vi "Daten zu cRIO.vi"   [LabVIEW 2020, in "Kommunikation mit PC.lvlib"]
uses:
  Kommunikation mit PC.lvlib
  Regler/Druckregler/Aktionen Param. Druckregler.ctl
  Allgemein/Aktionen FGV Dichtheitstest.ctl
  Allgemein/FGV Zustaende Aktionen.ctl
  Stoermeldungen/FGV Stoerungen Aktionen.ctl
  Verwaltung/FGV OUT Aktionen.ctl
  Allgemein/FGV FT-IR Kuehlung Aktionen.ctl
  Allgemein/Aktion FGV Klima.ctl
  Allgemein/Aktion FGV T90.ctl
  Allgemein/FGV Analysator aktiv.ctl
  Allgemein/Aktion FGV Zustandsbeleuchtung schalten.ctl
  Allgemein/Cluster Komm Systemeinstellungen.ctl
  Allgemein/Aktion FGV Komm Systemeinstellungen.ctl
  Konfig-Dateien/FGV Betriebsdaten Aktionen.ctl
  Konfig-Dateien/Aktionen Konfig.ctl
  Konfig-Dateien/Konfig-Dateien.lvlib
  Regler/Druckregler/Druckregler.lvlib
  Allgemein/Allgemein.lvlib
  Stoermeldungen/Stoermeldungen.lvlib
  Verwaltung/Verwaltung - cRIO.lvlib
  SysLog/SysLog_cRIO.lvlib
  CAN Interface/CAN Interface.lvlib
  CAN Interface/FGV CAN Daten Aktionen.ctl
  CAN Interface/Baude Rate.ctl
  Seiten/CAN Konfig/Konfig Daten PC.ctl
  Seiten/CAN Konfig/CAN Konfig.lvlib
types:
  T1 = typedef "Allgemein.lvlib/Aktion FGV Komm Systemeinstellungen.ctl" = enum16{"lesen", "schreiben"}
  T2 = typedef "Allgemein.lvlib/Cluster Komm Systemeinstellungen.ctl" = cluster{"ECO LNG":bool}
  T3 = typedef "Allgemein.lvlib/Aktion FGV Zustandsbeleuchtung schalten.ctl" = enum16{"lesen", "prüfen", "init", "Bit löschen", "ansteuern", "Aufheizphase"}
  T4 = typedef "Allgemein.lvlib/FGV Analysator aktiv.ctl" = enum16{"lesen", "Analysator", "CG Aufschaltung", "KAL Zustand", "AutaKal GT?"}
  T5 = typedef "Allgemein.lvlib/FGV Zustaende Aktionen.ctl" = enum16{"lesen", "Zustand PC", "Zustand cRIO", "Bildnummer", "Samplepoint", "Sysloglevel"}
  T6 = typedef "Allgemein.lvlib/Aktion FGV T90.ctl" = enum16{"lesen", "schreiben"}
  T7 = typedef "Allgemein.lvlib/Aktion FGV Klima.ctl" = enum16{"lesen", "Klimaanlage", "Container", "PNS"}
  T8 = typedef "Allgemein.lvlib/FGV FT-IR Kuehlung Aktionen.ctl" = enum16{"lesen", "Kühlung?"}
  T9 = typedef "Verwaltung - cRIO.lvlib/FGV OUT Aktionen.ctl" = enum16{"lesen", "ANA OUT", "DO 0-31", "DO 32-47"}
  T10 = typedef "Stoermeldungen.lvlib/FGV Stoerungen Aktionen.ctl" = enum16{"lesen", "Störung aktiv?", "1-64", "65-128"}
  T11 = typedef "Allgemein.lvlib/Aktionen FGV Dichtheitstest.ctl" = enum16{"lesen", "schreiben"}
  T12 = typedef "Regler.lvlib/Druckregler.lvlib/Aktionen Param. Druckregler.ctl" = enum16{"lesen", "schreiben", "Regler FT-IR", "Regler Ausgang", "Regler Durchfluss", "Regler PMA", "Regler NDIR", "Regler Filterblock", "Regler Gaskühler", "Regler Kalter Block"}
  T13 = typedef "Bildwechsel.lvlib/Bild-Auswahl.ctl" = enum16{"lesen", "Initialisieren", "Beenden", "Grafik", "Anlagenübersicht", "Anlagengrenzwerte", "Log Konfig", "Gaszuordnung AO", "Erw. Konfiguration", "FT-IR  ", "Störmeldungen", "Störmeldepuffer", "Störmeldekonfig", "PNS Grenzwerte", "Statusübersicht", "Linearisierung", "ARN", "EPA Dichtheitstest", "FID", "PMA", "CalGas", "Lambda", "Interference", "Amium PNS", "EPA T90", "Interference N2O", "Scheduler", "Systemeinstellungen", "EPA Drift", "CAN Konfig"}
  T14 = cluster{"SysLogLevel":u16, "Software Version":string}
  T15 = cluster{"Numeric":u16, "Numeric":u16, "Numeric":u16, "Numeric":u16, "Numeric":u16}
  T16 = cluster{"Numeric":u16, "Numeric":u16, "Numeric":u16}
  T17 = cluster{"Boolean":bool, "Boolean":bool, "Boolean":bool}
  T18 = typedef "Konfig-Dateien.lvlib/FGV Betriebsdaten Aktionen.ctl" = enum16{"lesen", "Anlagengrenzw.", "PID Param.", "Sonstige", "Sensor Para."}
  T19 = typedef "Konfig-Dateien.lvlib/Aktionen Konfig.ctl" = enum16{"lesen", "laden", "speichern  System.ini", "speichern Anlagengrenzw.", "speichern PID + Sonstige", "speichern BSZ BMP", "speichern BSZ FT-IR", "speichern Stickstoff Bef.", "speichern Ext. Stickstoff Bef.", "speichern CAN_Konfig"}
  T20 = typedef "CAN Konfig.lvlib/Konfig Daten PC.ctl" = cluster{"Baude Rate":T21, "COM state":u8, "Frame-ID FTIR Start":u32, "Frame-ID FTIR End":u32, "Frame-ID Status Start":u32, "Frame-ID Status End":u32, "Zustand Information":u32, "Aktion":u32, "Frame-ID FTIR Arry":u32[], "Frame-ID Status Arry":u32[], "GPS Start":u32, "Interface":refnum<k21>}
  T21 = typedef "CAN Interface.lvlib/Baude Rate.ctl" = u32
  T22 = typedef "CAN Interface.lvlib/FGV CAN Daten Aktionen.ctl" = enum16{"lesen", "Daten", "Konfig", "laden", "speichern", "Status"}
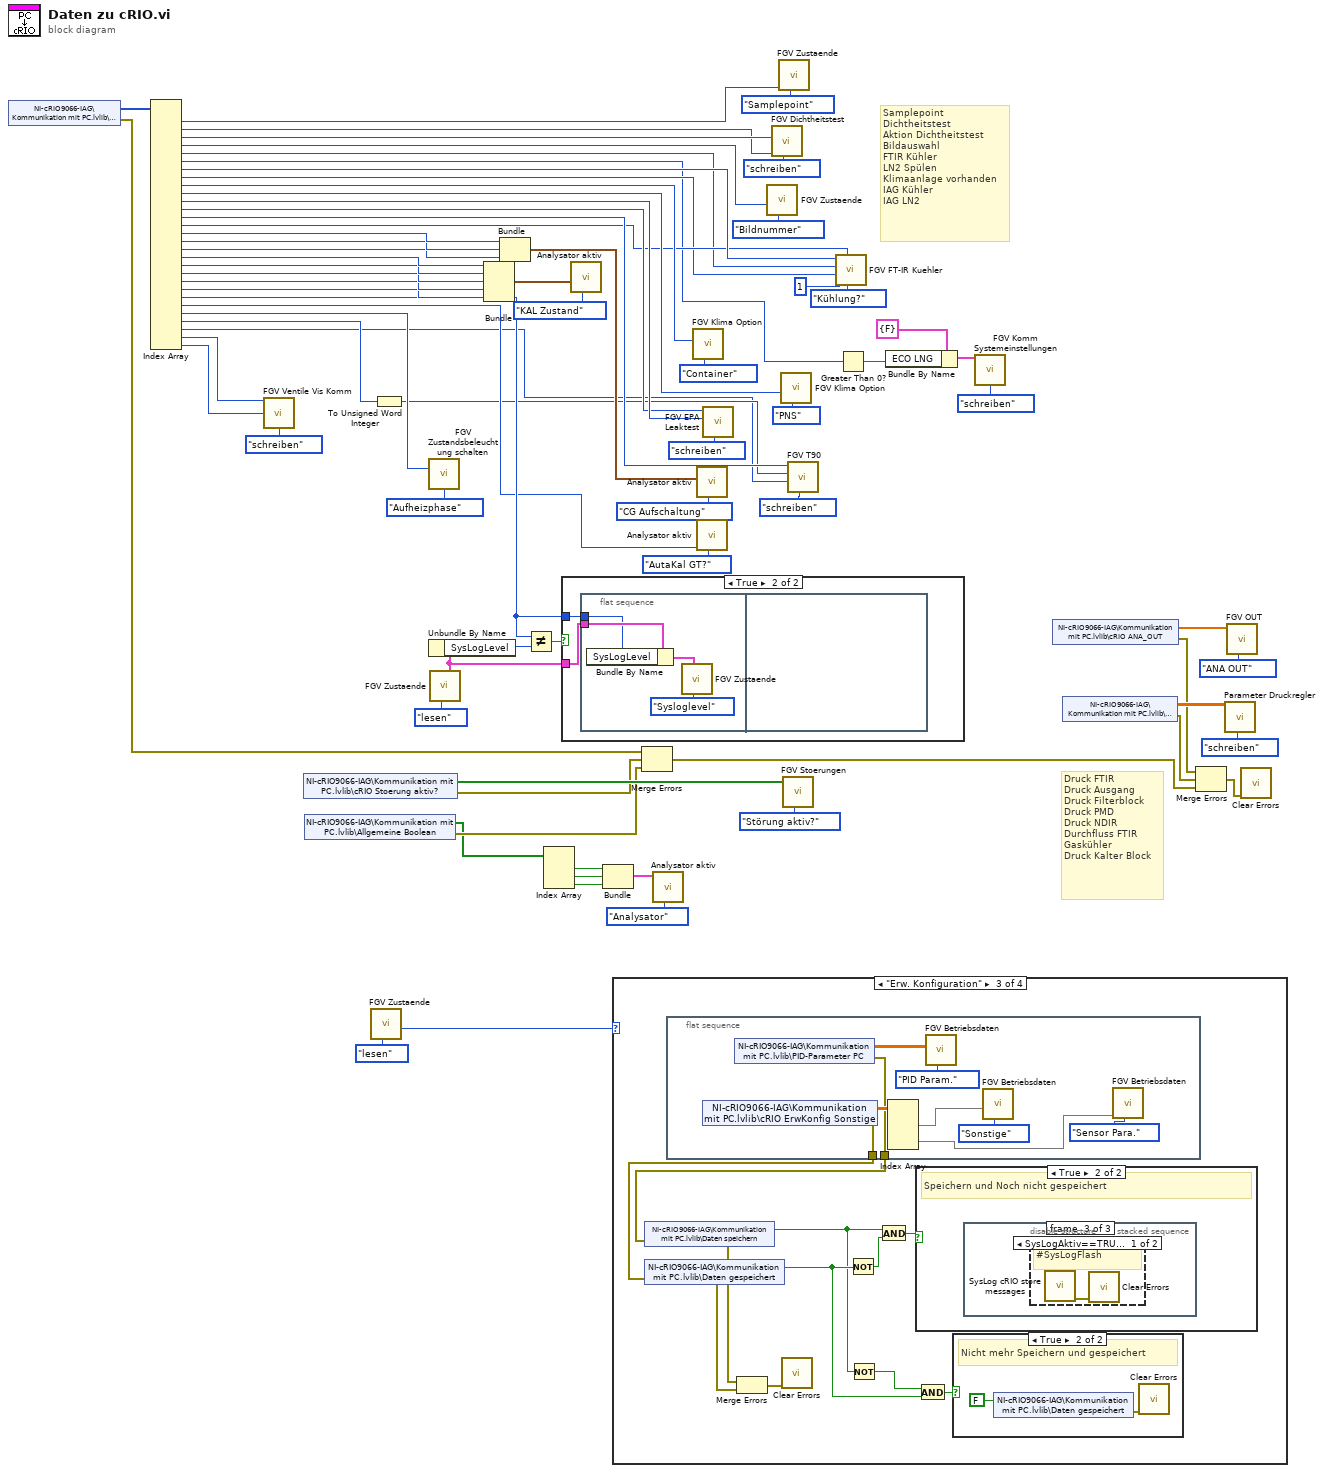
[diagram p0: block diagram]
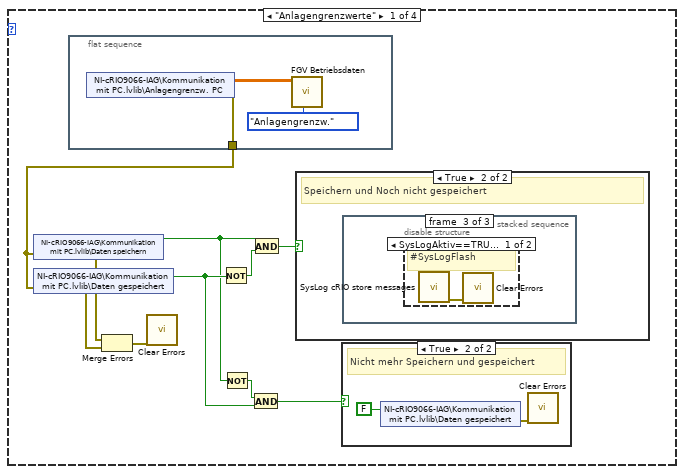
[diagram p3: hidden frame]
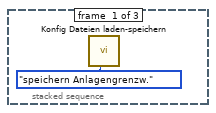
[diagram p6: hidden frame]
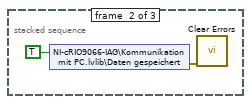
[diagram p7: hidden frame]
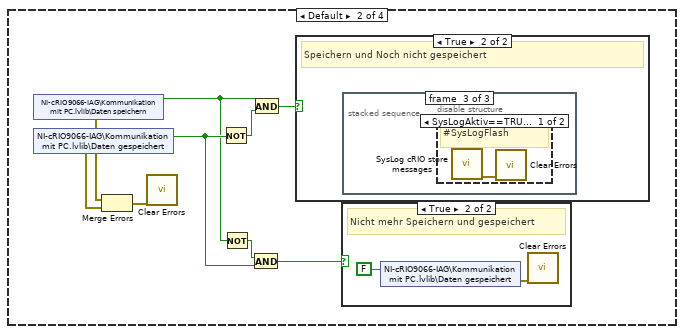
[diagram p9: hidden frame]
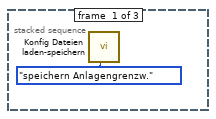
[diagram p12: hidden frame]
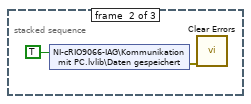
[diagram p13: hidden frame]
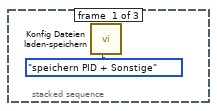
[diagram p17: hidden frame]
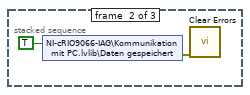
[diagram p18: hidden frame]
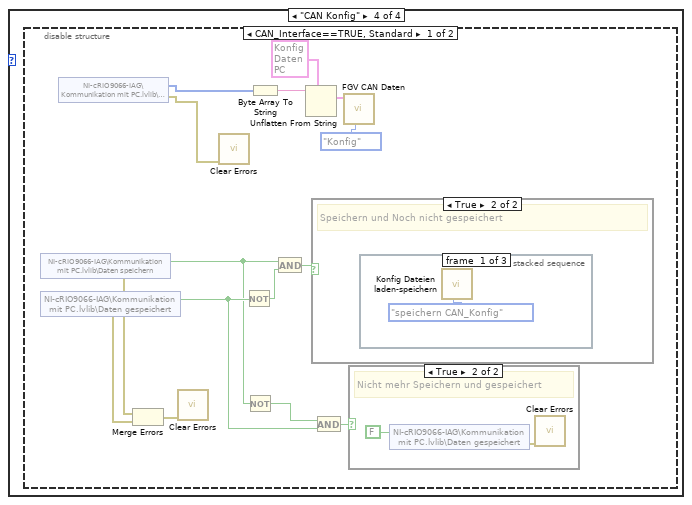
[diagram p20: hidden frame]
diagram:
  # "Druck FTIR\nDruck Ausgang\nDruck Filterblock\nDruck PMD\nDruck NDIR\nDurchfluss FTIR\nGaskühler\nDruck Kalter Block"
  # "Samplepoint\nDichtheitstest\nAktion Dichtheitstest\nBildauswahl\nFTIR Kühler \nLN2 Spülen\nKlimaanlage vorhanden\nIAG Kühler\nIAG LN2"
  n1 = shared-variable "NI-cRIO9066-IAG\\Kommunikation mit PC.lvlib\\Samplepoint"() -> (w74:u16[], error out=w60:errorcluster)  [unwired: 1 in]
  n2 = Index Array(array=w74) -> (element #1=w11:u16, element #2=w12:u16, element #3=w13:u16, element #4=w14:u16, element #5=w15:u16, element #6=w5:u16, element #7=w55:u16, element #8=w9:u16, element #9=w56:u16, element #10=w54:u16, element #11=w51:u16, element #12=w50:u16, element #13=w48:u16, element #14=w47:u16, element #15=w46:u16, element #16=w45:u16, element #17=w44:u16, element #18=w43:u16, element #19=w42:u16, element #20=w41:u16, element #21=w40:u16, element #22=w28:u16, element #23=w24:u16, element #24=w21:u16, element #25=w19:u16, element #26=w18:u16, element #27=w10:u16, element #28=w1:u16, element #29=w2:u16)  [unwired: 29 in]
  n3 = call "FGV Ventile Vis Komm.vi"("Ventile schalten"=w1, "Betrieb"=w2, "Aktion"=enum16{"lesen", "schreiben"}."schreiben") -> ()  [unwired: 10 in, 3 out]
  n4 = shared-variable "NI-cRIO9066-IAG\\Kommunikation mit PC.lvlib\\cRIO Stoerung aktiv?"() -> (w64:bool[], error out=w61:errorcluster)  [unwired: 1 in]
  n5 = shared-variable "NI-cRIO9066-IAG\\Kommunikation mit PC.lvlib\\Allgemeine Boolean"() -> (w34:bool[], error out=w35:errorcluster)  [unwired: 1 in]
  n6 = call "FGV Zustaende.vi"("Aktionen"=FGV_Zustaende_Aktionen."lesen") -> ("aktuelle Bildnummer"=w66:T13)  [unwired: 6 in, 4 out]
  n7 = To Unsigned Word Integer(number=w18) -> (unsigned 16bit integer=w17:u16)
  n8 = call "FGV Zustandsbeleuchtung schalten.vi"("Aufheizphase"=w19, "Aktion"=Aktion_FGV_Zustandsbeleuchtung_schalten."Aufheizphase") -> ()  [unwired: 12 in, 2 out]
  n9 = call "FGV Zustaende.vi"("Aktionen"=FGV_Zustaende_Aktionen."lesen") -> ("SL SV Cluster"=w23:T14)  [unwired: 6 in, 4 out]
  n10 = Unbundle By Name(w23) -> ("SysLogLevel"=w26:u16)
  n11 = Bundle("Numeric"=w43, "Numeric"=w42, "Numeric"=w41, "Numeric"=w40, "Numeric"=w28) -> (w36:T15)  [unwired: 1 in]
  n12 = Bundle("Numeric"=w46, "Numeric"=w45, "Numeric"=w44) -> (w38:T16)  [unwired: 1 in]
  n13 = Not Equal?(x=w24, y=w26) -> (x != y?=w25:bool)
  n14 = Index Array(array=w34) -> (element #1=w33:bool, element #2=w32:bool, element #3=w31:bool)  [unwired: 3 in]
  n15 = case shown="True" w25 {
    tunnel: w24 -> [_ w77]
    tunnel: w23 -> [_ w78]
    frame False {
    }
    frame True {
      n16 = flat-sequence {
        tunnel: w78 -> [w81]
        tunnel: w77 -> [w80]
        frame #0 {
          n17 = Bundle By Name(cluster=w81, "SysLogLevel"=w80) -> (w79:T14)
          n18 = call "FGV Zustaende.vi"("Aktionen"=FGV_Zustaende_Aktionen."Sysloglevel", "SL SV Cluster"=w79) -> ()  [unwired: 5 in, 5 out]
        }
        frame #1 {
        }
      }
    }
  }
  n19 = call "Analysator aktiv.vi"("Aktion"=FGV_Analysator_aktiv."KAL Zustand", "Kalibrieren"=w36) -> ()  [unwired: 6 in, 4 out]
  n20 = Bundle("Boolean"=w33, "Boolean"=w32, "Boolean"=w31) -> (w29:T17)  [unwired: 1 in]
  n21 = case shown="\"Erw. Konfiguration\"" w66 {
    frame "Anlagengrenzwerte" {
      n22 = shared-variable "NI-cRIO9066-IAG\\Kommunikation mit PC.lvlib\\Daten speichern"(error in=w83) -> (w88:bool, error out=w85:errorcluster)
      n23 = shared-variable "NI-cRIO9066-IAG\\Kommunikation mit PC.lvlib\\Daten gespeichert"(error in=w83) -> (w89:bool, error out=w84:errorcluster)
      n24 = flat-sequence {
        tunnel: [w94] -> w83
        frame #0 {
          n25 = shared-variable "NI-cRIO9066-IAG\\Kommunikation mit PC.lvlib\\Anlagengrenzw. PC"() -> (w93:sgl[][], error out=w94:errorcluster)  [unwired: 1 out]
          n26 = call "FGV Betriebsdaten.vi"("Aktionen"=FGV_Betriebsdaten_Aktionen."Anlagengrenzw.", "Anlagen-Grenzwerte"=w93) -> ()  [unwired: 6 in, 4 out]
        }
      }
      n27 = Merge Errors(w85, w84) -> (w86:errorcluster)
      n28 = call <vilib>:"Clear Errors.vi"("error in (no error)"=w86) -> ()  [unwired: 5 in, 2 out]
      n29 = Not(x=w89) -> (.not. x?=w92:bool)
      n30 = Not(x=w88) -> (.not. x?=w87:bool)
      n31 = And(x=w87, y=w89) -> (x .and. y?=w90:bool)
      n32 = And(x=w88, y=w92) -> (x .and. y?=w91:bool)
      n33 = case shown="True" w91 {
        frame False {
        }
        frame True {
          # "Speichern und Noch nicht gespeichert"
          n34 = stacked-sequence {
            frame #0 {
              n35 = call "Konfig Dateien laden-speichern.vi"("Aktion"=Aktionen_Konfig."speichern Anlagengrenzw.") -> ()  [unwired: 10 in, 1 out]
            }
            frame #1 {
              n36 = shared-variable "NI-cRIO9066-IAG\\Kommunikation mit PC.lvlib\\Daten gespeichert"(TRUE ("Daten gespeichert")) -> (error out=w99:errorcluster)  [unwired: 1 in]
              n37 = call <vilib>:"Clear Errors.vi"("error in (no error)"=w99) -> ()  [unwired: 5 in, 2 out]
            }
            frame #2 {
              n38 = disable-structure shown="SysLogAktiv==TRUE" {
                frame condition #0 (active) {
                  # "#SysLogFlash"
                  n39 = call "SysLog cRIO store messages.vi"() -> ("Fehler (out)"=w101:errorcluster)  [unwired: 11 in]
                  n40 = call <vilib>:"Clear Errors.vi"("error in (no error)"=w101) -> ()  [unwired: 5 in, 2 out]
                }
                frame condition #1 {
                }
              }
            }
          }
        }
      }
      n41 = case shown="True" w90 {
        frame False {
        }
        frame True {
          # "Nicht mehr Speichern und gespeichert"
          n42 = shared-variable "NI-cRIO9066-IAG\\Kommunikation mit PC.lvlib\\Daten gespeichert"(FALSE ("Daten gespeichert")) -> (error out=w96:errorcluster)  [unwired: 1 in]
          n43 = call <vilib>:"Clear Errors.vi"("error in (no error)"=w96) -> ()  [unwired: 5 in, 2 out]
        }
      }
    }
    frame Default {
      n44 = shared-variable "NI-cRIO9066-IAG\\Kommunikation mit PC.lvlib\\Daten speichern"() -> (w106:bool, error out=w103:errorcluster)  [unwired: 1 in]
      n45 = shared-variable "NI-cRIO9066-IAG\\Kommunikation mit PC.lvlib\\Daten gespeichert"() -> (w107:bool, error out=w102:errorcluster)  [unwired: 1 in]
      n46 = Merge Errors(w103, w102) -> (w104:errorcluster)
      n47 = call <vilib>:"Clear Errors.vi"("error in (no error)"=w104) -> ()  [unwired: 5 in, 2 out]
      n48 = Not(x=w107) -> (.not. x?=w110:bool)
      n49 = Not(x=w106) -> (.not. x?=w105:bool)
      n50 = And(x=w105, y=w107) -> (x .and. y?=w108:bool)
      n51 = And(x=w106, y=w110) -> (x .and. y?=w109:bool)
      n52 = case shown="True" w109 {
        frame False {
        }
        frame True {
          # "Speichern und Noch nicht gespeichert"
          n53 = stacked-sequence {
            frame #0 {
              n54 = call "Konfig Dateien laden-speichern.vi"("Aktion"=Aktionen_Konfig."speichern Anlagengrenzw.") -> ()  [unwired: 10 in, 1 out]
            }
            frame #1 {
              n55 = shared-variable "NI-cRIO9066-IAG\\Kommunikation mit PC.lvlib\\Daten gespeichert"(TRUE ("Daten gespeichert")) -> (error out=w114:errorcluster)  [unwired: 1 in]
              n56 = call <vilib>:"Clear Errors.vi"("error in (no error)"=w114) -> ()  [unwired: 5 in, 2 out]
            }
            frame #2 {
              n57 = disable-structure shown="SysLogAktiv==TRUE" {
                frame condition #0 (active) {
                  # "#SysLogFlash"
                  n58 = call "SysLog cRIO store messages.vi"() -> ("Fehler (out)"=w116:errorcluster)  [unwired: 11 in]
                  n59 = call <vilib>:"Clear Errors.vi"("error in (no error)"=w116) -> ()  [unwired: 5 in, 2 out]
                }
                frame condition #1 {
                }
              }
            }
          }
        }
      }
      n60 = case shown="True" w108 {
        frame False {
        }
        frame True {
          # "Nicht mehr Speichern und gespeichert"
          n61 = shared-variable "NI-cRIO9066-IAG\\Kommunikation mit PC.lvlib\\Daten gespeichert"(FALSE ("Daten gespeichert")) -> (error out=w111:errorcluster)  [unwired: 1 in]
          n62 = call <vilib>:"Clear Errors.vi"("error in (no error)"=w111) -> ()  [unwired: 5 in, 2 out]
        }
      }
    }
    frame "Erw. Konfiguration" {
      n63 = shared-variable "NI-cRIO9066-IAG\\Kommunikation mit PC.lvlib\\Daten speichern"(error in=w117) -> (w123:bool, error out=w120:errorcluster)
      n64 = shared-variable "NI-cRIO9066-IAG\\Kommunikation mit PC.lvlib\\Daten gespeichert"(error in=w118) -> (w124:bool, error out=w119:errorcluster)
      n65 = flat-sequence {
        tunnel: [w132] -> w118
        tunnel: [w131] -> w117
        frame #0 {
          n66 = shared-variable "NI-cRIO9066-IAG\\Kommunikation mit PC.lvlib\\cRIO ErwKonfig Sonstige"() -> (w133:sgl[][], error out=w132:errorcluster)  [unwired: 1 in]
          n67 = shared-variable "NI-cRIO9066-IAG\\Kommunikation mit PC.lvlib\\PID-Parameter PC"() -> (w135:sgl[][], error out=w131:errorcluster)  [unwired: 1 out]
          n68 = Index Array(array=w133) -> (element #1=w130:sgl[], element #2=w128:sgl[])  [unwired: 4 in]
          n69 = call "FGV Betriebsdaten.vi"("Aktionen"=FGV_Betriebsdaten_Aktionen."PID Param.", "PID-Parameter"=w135) -> ()  [unwired: 6 in, 4 out]
          n70 = call "FGV Betriebsdaten.vi"("Aktionen"=FGV_Betriebsdaten_Aktionen."Sonstige", "Sonstige"=w130) -> ()  [unwired: 6 in, 4 out]
          n71 = call "FGV Betriebsdaten.vi"("Aktionen"=FGV_Betriebsdaten_Aktionen."Sensor Para.", "Parameter Sensoren"=w128) -> ()  [unwired: 6 in, 4 out]
        }
      }
      n72 = Merge Errors(w120, w119) -> (w121:errorcluster)
      n73 = call <vilib>:"Clear Errors.vi"("error in (no error)"=w121) -> ()  [unwired: 5 in, 2 out]
      n74 = Not(x=w124) -> (.not. x?=w127:bool)
      n75 = Not(x=w123) -> (.not. x?=w122:bool)
      n76 = And(x=w123, y=w127) -> (x .and. y?=w126:bool)
      n77 = case shown="True" w126 {
        frame False {
        }
        frame True {
          # "Speichern und Noch nicht gespeichert"
          n78 = stacked-sequence {
            frame #0 {
              n79 = call "Konfig Dateien laden-speichern.vi"("Aktion"=Aktionen_Konfig."speichern PID + Sonstige") -> ()  [unwired: 10 in, 1 out]
            }
            frame #1 {
              n80 = shared-variable "NI-cRIO9066-IAG\\Kommunikation mit PC.lvlib\\Daten gespeichert"(TRUE ("Daten gespeichert")) -> (error out=w140:errorcluster)  [unwired: 1 in]
              n81 = call <vilib>:"Clear Errors.vi"("error in (no error)"=w140) -> ()  [unwired: 5 in, 2 out]
            }
            frame #2 {
              n82 = disable-structure shown="SysLogAktiv==TRUE" {
                frame condition #0 (active) {
                  # "#SysLogFlash"
                  n83 = call "SysLog cRIO store messages.vi"() -> ("Fehler (out)"=w142:errorcluster)  [unwired: 11 in]
                  n84 = call <vilib>:"Clear Errors.vi"("error in (no error)"=w142) -> ()  [unwired: 5 in, 2 out]
                }
                frame condition #1 {
                }
              }
            }
          }
        }
      }
      n85 = And(x=w122, y=w124) -> (x .and. y?=w125:bool)
      n86 = case shown="True" w125 {
        frame False {
        }
        frame True {
          # "Nicht mehr Speichern und gespeichert"
          n87 = shared-variable "NI-cRIO9066-IAG\\Kommunikation mit PC.lvlib\\Daten gespeichert"(FALSE ("Daten gespeichert")) -> (error out=w137:errorcluster)  [unwired: 1 in]
          n88 = call <vilib>:"Clear Errors.vi"("error in (no error)"=w137) -> ()  [unwired: 5 in, 2 out]
        }
      }
    }
    frame "CAN Konfig" {
      n89 = disable-structure shown="CAN_Interface==TRUE, Standard" {
        frame condition #0 {
          n90 = shared-variable "NI-cRIO9066-IAG\\Kommunikation mit PC.lvlib\\Daten speichern"() -> (w153:bool, error out=w150:errorcluster)  [unwired: 1 in]
          n91 = shared-variable "NI-cRIO9066-IAG\\Kommunikation mit PC.lvlib\\Daten gespeichert"() -> (w154:bool, error out=w149:errorcluster)  [unwired: 1 in]
          n92 = shared-variable "NI-cRIO9066-IAG\\Kommunikation mit PC.lvlib\\CAN_Konfig"() -> (w144:u8[], error out=w143:errorcluster)  [unwired: 1 in]
          n93 = Merge Errors(w150, w149) -> (w151:errorcluster)
          n94 = call <vilib>:"Clear Errors.vi"("error in (no error)"=w151) -> ()  [unwired: 5 in, 2 out]
          n95 = call <vilib>:"Clear Errors.vi"("error in (no error)"=w143) -> ()  [unwired: 5 in, 2 out]
          n96 = Not(x=w154) -> (.not. x?=w157:bool)
          n97 = Not(x=w153) -> (.not. x?=w152:bool)
          n98 = Byte Array To String(unsigned byte array=w144) -> (string=w148:string)
          n99 = And(x=w153, y=w157) -> (x .and. y?=w156:bool)
          n100 = Unflatten From String(type=T20 {"Baude Rate"=250000, "COM state"=144, "Frame-ID FTIR Start"=0, "Frame-ID FTIR End"=0, "Frame-ID Status Start"=0, "Frame-ID Status End"=0, "Zustand Information"=0, "Aktion"=0, "Frame-ID FTIR Arry"=[], "Frame-ID Status Arry"=[], "GPS Start"=0, "Interface"="CAN1"} ("Konfig Daten 2"), binary string=w148) -> (value=w146:T20)  [unwired: 3 in, 2 out]
          n101 = case shown="True" w156 {
            frame False {
            }
            frame True {
              # "Speichern und Noch nicht gespeichert"
              n102 = stacked-sequence {
                frame #0 {
                  n103 = call "Konfig Dateien laden-speichern.vi"("Aktion"=Aktionen_Konfig."speichern CAN_Konfig") -> ()  [unwired: 10 in, 1 out]
                }
                frame #1 {
                  n104 = shared-variable "NI-cRIO9066-IAG\\Kommunikation mit PC.lvlib\\Daten gespeichert"(TRUE ("Daten gespeichert")) -> (error out=w161:errorcluster)  [unwired: 1 in]
                  n105 = call <vilib>:"Clear Errors.vi"("error in (no error)"=w161) -> ()  [unwired: 5 in, 2 out]
                }
                frame #2 {
                  n106 = disable-structure shown="SysLogAktiv==TRUE" {
                    frame condition #0 (active) {
                      # "#SysLogFlash"
                      n107 = call "SysLog cRIO store messages.vi"() -> ("Fehler (out)"=w163:errorcluster)  [unwired: 11 in]
                      n108 = call <vilib>:"Clear Errors.vi"("error in (no error)"=w163) -> ()  [unwired: 5 in, 2 out]
                    }
                    frame condition #1 {
                    }
                  }
                }
              }
            }
          }
          n109 = And(x=w152, y=w154) -> (x .and. y?=w155:bool)
          n110 = call "FGV CAN Daten.vi"("Aktionen"=FGV_CAN_Daten_Aktionen."Konfig", "Konfig Daten 2"=w146) -> ()  [unwired: 7 in, 3 out]
          n111 = case shown="True" w155 {
            frame False {
            }
            frame True {
              # "Nicht mehr Speichern und gespeichert"
              n112 = shared-variable "NI-cRIO9066-IAG\\Kommunikation mit PC.lvlib\\Daten gespeichert"(FALSE ("Daten gespeichert")) -> (error out=w158:errorcluster)  [unwired: 1 in]
              n113 = call <vilib>:"Clear Errors.vi"("error in (no error)"=w158) -> ()  [unwired: 5 in, 2 out]
            }
          }
        }
        frame condition #1 (active) {
        }
      }
    }
  }
  n114 = Merge Errors(w60, w61, w35) -> (w59:errorcluster)
  n115 = call "Analysator aktiv.vi"("Aktion"=FGV_Analysator_aktiv."Analysator", "Status Analysatoren"=w29) -> ()  [unwired: 6 in, 4 out]
  n116 = call "FGV Klima Option.vi"("Aktion"=Aktion_FGV_Klima."Container", "Container"=w56) -> ()  [unwired: 7 in, 3 out]
  n117 = call "Analysator aktiv.vi"("Aktion"=FGV_Analysator_aktiv."CG Aufschaltung", "Aufschaltung CalGas"=w38) -> ()  [unwired: 6 in, 4 out]
  n118 = call "Analysator aktiv.vi"("Aktion"=FGV_Analysator_aktiv."AutaKal GT?", "Autokal GT?"=w21) -> ()  [unwired: 6 in, 4 out]
  n119 = call "FGV EPA Leaktest.vi"("Aktion"=enum16{"lesen", "schreiben"}."schreiben", "Leaktest aktiv"=w51, "Leaktest Zustand"=w50) -> ()  [unwired: 7 in, 2 out]
  n120 = call "FGV Zustaende.vi"("Aktionen"=FGV_Zustaende_Aktionen."Bildnummer", "aktuelle Bildnummer"=w14) -> ()  [unwired: 5 in, 5 out]
  n121 = call "FGV Dichtheitstest.vi"("Aktionen"=Aktionen_FGV_Dichtheitstest."schreiben", "Dichtheitstest?"=w12, "Aktionen Dichtheitstest"=w13) -> ()  [unwired: 7 in, 2 out]
  n122 = call "FGV Zustaende.vi"("Aktionen"=FGV_Zustaende_Aktionen."Samplepoint", "Samplepoint"=w11) -> ()  [unwired: 5 in, 5 out]
  n123 = call "FGV Klima Option.vi"("Aktion"=Aktion_FGV_Klima."PNS", "PNS vorhanden"=w54) -> ()  [unwired: 7 in, 3 out]
  n124 = call "FGV Stoerungen.vi"("Aktionen"=FGV_Stoerungen_Aktionen."Störung aktiv?", "Störung aktiv?"=w64) -> ()  [unwired: 7 in, 3 out]
  n125 = call "FGV T90.vi"("Aktion"=Aktion_FGV_T90."schreiben", "Entnahme aktiv"=w10, "N2 Spülen aktiv"=w17, "T90 aktiv"=w48) -> ()  [unwired: 4 in, 4 out]
  n126 = call "FGV FT-IR Kuehler.vi"("Aktionen"=FGV_FT-IR_Kuehlung_Aktionen."Kühlung?", "N2 zu PNS"=w47, "FT-IR Kühler"=u16 1, "Durchflusssensor 0-5V"=w9, "LN2 Spülen"=w15, "mit GN2 spülen"=w55) -> ()  [unwired: 1 in, 5 out]
  n127 = Greater Than 0?(x=w5) -> (x > 0?=w6:bool)
  n128 = Bundle By Name(cluster=T2 {"ECO LNG"=FALSE} ("Systemeinstellungen"), "ECO LNG"=w6) -> (w7:T2)
  n129 = call "FGV Komm Systemeinstellungen.vi"("Systemeinstellungen"=w7, "Aktion"=Aktion_FGV_Komm_Systemeinstellungen."schreiben") -> ()  [unwired: 12 in, 2 out]
  n130 = shared-variable "NI-cRIO9066-IAG\\Kommunikation mit PC.lvlib\\cRIO ANA_OUT"() -> (w62:sgl[], error out=w71:errorcluster)  [unwired: 1 in]
  n131 = shared-variable "NI-cRIO9066-IAG\\Kommunikation mit PC.lvlib\\Param.Regler"() -> (w75:sgl[][], error out=w70:errorcluster)  [unwired: 1 in]
  n132 = Merge Errors(w71, w70, w59) -> (w72:errorcluster)
  n133 = call "Parameter Druckregler.vi"("Regelparameter"=w75, "Aktionen"=Aktionen_Param._Druckregler."schreiben") -> ()  [unwired: 9 in, 9 out]
  n134 = call "FGV OUT.vi"("Aktion"=FGV_OUT_Aktionen."ANA OUT", "ANA OUT"=w62) -> ()  [unwired: 6 in, 4 out]
  n135 = call <vilib>:"Clear Errors.vi"("error in (no error)"=w72) -> ()  [unwired: 5 in, 2 out]
